vi "Create 1D Table.vi"(4 "use apostrophes (F)":bool, 5 "column vector (F)":bool, 8 "formatted values":string[](array[string]), 11 "table name":string) -> (0 "can be indented?":bool, 3 "table":string)   [LabVIEW 2013, in "infolib.lvlib"]
doc: "Generates 1D table - row or column."
uses:
  infolib.lvlib
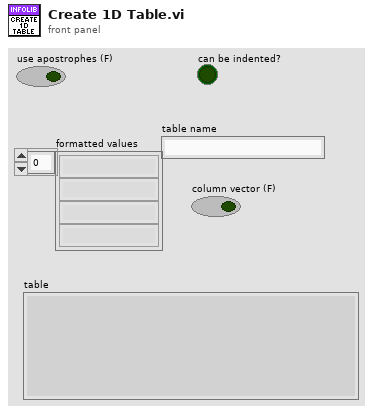
[diagram p1: front panel]
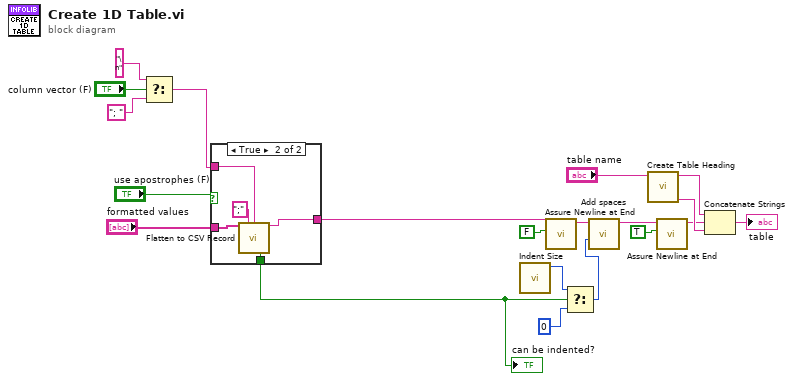
[diagram p0: block diagram]
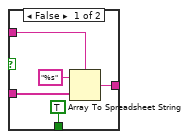
[diagram p2: hidden frame]
diagram:
  n1 = Select(t="\n" ("delimiter (Tab)"), s="column vector (F)", f="; " ("delimiter (Tab)")) -> (s? t:f=w1:string)
  n2 = case shown="True" "use apostrophes (F)" {
    tunnel: "formatted values" -> [w25 w30]
    tunnel: [w24 w29] -> w5
    tunnel: w1 -> [w22 w27]
    tunnel: [TRUE ("can be indented?") w28] -> w7
    frame False {
      n3 = Array To Spreadsheet String(delimiter (Tab)=w22, array=w25, 3:"%s" ("format string")) -> (spreadsheet string=w24:string)
    }
    frame True {
      n4 = call "Flatten to CSV Record.vi"("row of strings"=w30, "protected symbol (,)"=";", "item separator (empty - use protected symbol)"=w27) -> ("can be indented?"=w28:bool, "CSV record"=w29:string)  [unwired: 10 in, 1 out]
    }
  }
  "can be indented?" <- w7
  n5 = call "Indent Size.vi"() -> ("indent size"=w10:i32)  [unwired: 10 in, 1 out]
  n6 = call "Assure Newline at End.vi"("Set End Of Line (F)"=FALSE, "string"=w5) -> ("string out"=w16:string)  [unwired: 9 in]
  n7 = Select(t=w10, s=w7, f=0) -> (s? t:f=w9:i32)
  n8 = call "Add spaces.vi"("spaces no"=w9, "input string"=w16) -> ("result string"=w14:string)  [unwired: 9 in]
  n9 = call "Create Table Heading.vi"("table name"="table name") -> ("table end"=w18:string, "table start"=w19:string)  [unwired: 9 in]
  n10 = call "Assure Newline at End.vi"("Set End Of Line (F)"=TRUE, "string"=w14) -> ("string out"=w13:string)  [unwired: 9 in]
  n11 = Concatenate Strings(w19, w13, w18) -> (→"table":string)
